vi "LabView SMART BABY CARE .vi"() -> ()   [LabVIEW 2020]
uses:
  <vilib>/Instr/_visa.llb/VISA Configure Serial Port (Instr).vi
  <vilib>/express/express analysis/Spectral/Block/exnSpectralBlock spectral measurements peak poly.vi
  <vilib>/express/express analysis/Spectral/Block/exnSpectralBlock spectral measurements peak DDT.vi
  <vilib>/httpClient/PUTBuffer.vi
  <vilib>/express/express analysis/Spectral/XNode/ExpressSpectralMeasurementsBlockNode.xnode
  <vilib>/httpClient/LabVIEWHTTPClient.lvlib
  <vilib>/ptbypt/NI_PtbyPt.lvlib
panel:
  out "reset signal":bool caption="Time has Elapsed"
  out "swing status":bool caption="Time has Elapsed"
  out "net status":bool caption="Time has Elapsed"
  out "fan status":bool caption="Time has Elapsed"
  out "fan speed":dbl
  out "temperture":dbl(knob) scale=15.0..50.0
  in  "VISA resource name":refnum<visa-resource-name>
  out "danger_movement":bool caption="Time has Elapsed"
  out "angle":dbl(knob) scale=-90.0..90.0
  out "vol-angle":dbl
  out "crying_sound":bool caption="Time has Elapsed"
  out "baby_present":bool
  out "lux":dbl
  out "volt lux":dbl
  out "volt wet":dbl
  out "wet":bool caption="Time has Elapsed"
  out "Waveform Graph":dynamicdata(graph)
  out "baby_crying":bool caption="Time has Elapsed"
  out "Amplitude of sound":dbl
  out "net comand":bool
  out "fan command":bool
  in  "stop":bool
  # "SMART BABY CARE SYSTEM"
  # "BY GROUP 05"
  # "BABY MONITORING AND CRY DETECT"
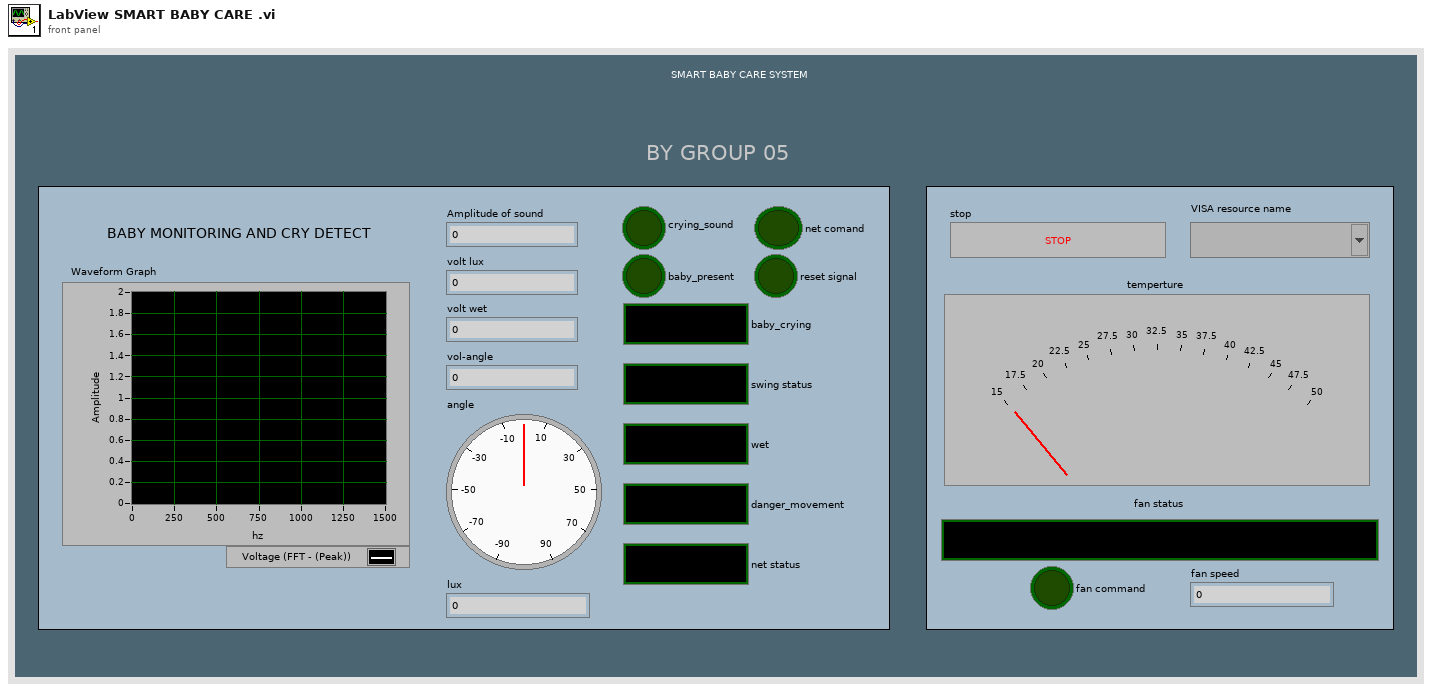
[diagram p1: front panel]
types:
  T1 = typedef "LabVIEWHTTPClient.lvlib/ClientHandle.ctl" = refnum<k1>
  T2 = cluster{"fan_command":bool, "net_command":bool, "net_adjust_time":string, "net_reset":bool}
  T3 = cluster{"averaging mode":u16, "weighting mode":u16, "number of averages":u32}
  T4 = cluster{"dB On (F)":bool, "unwrap phase (F)":bool, "convert to degree (F)":bool}
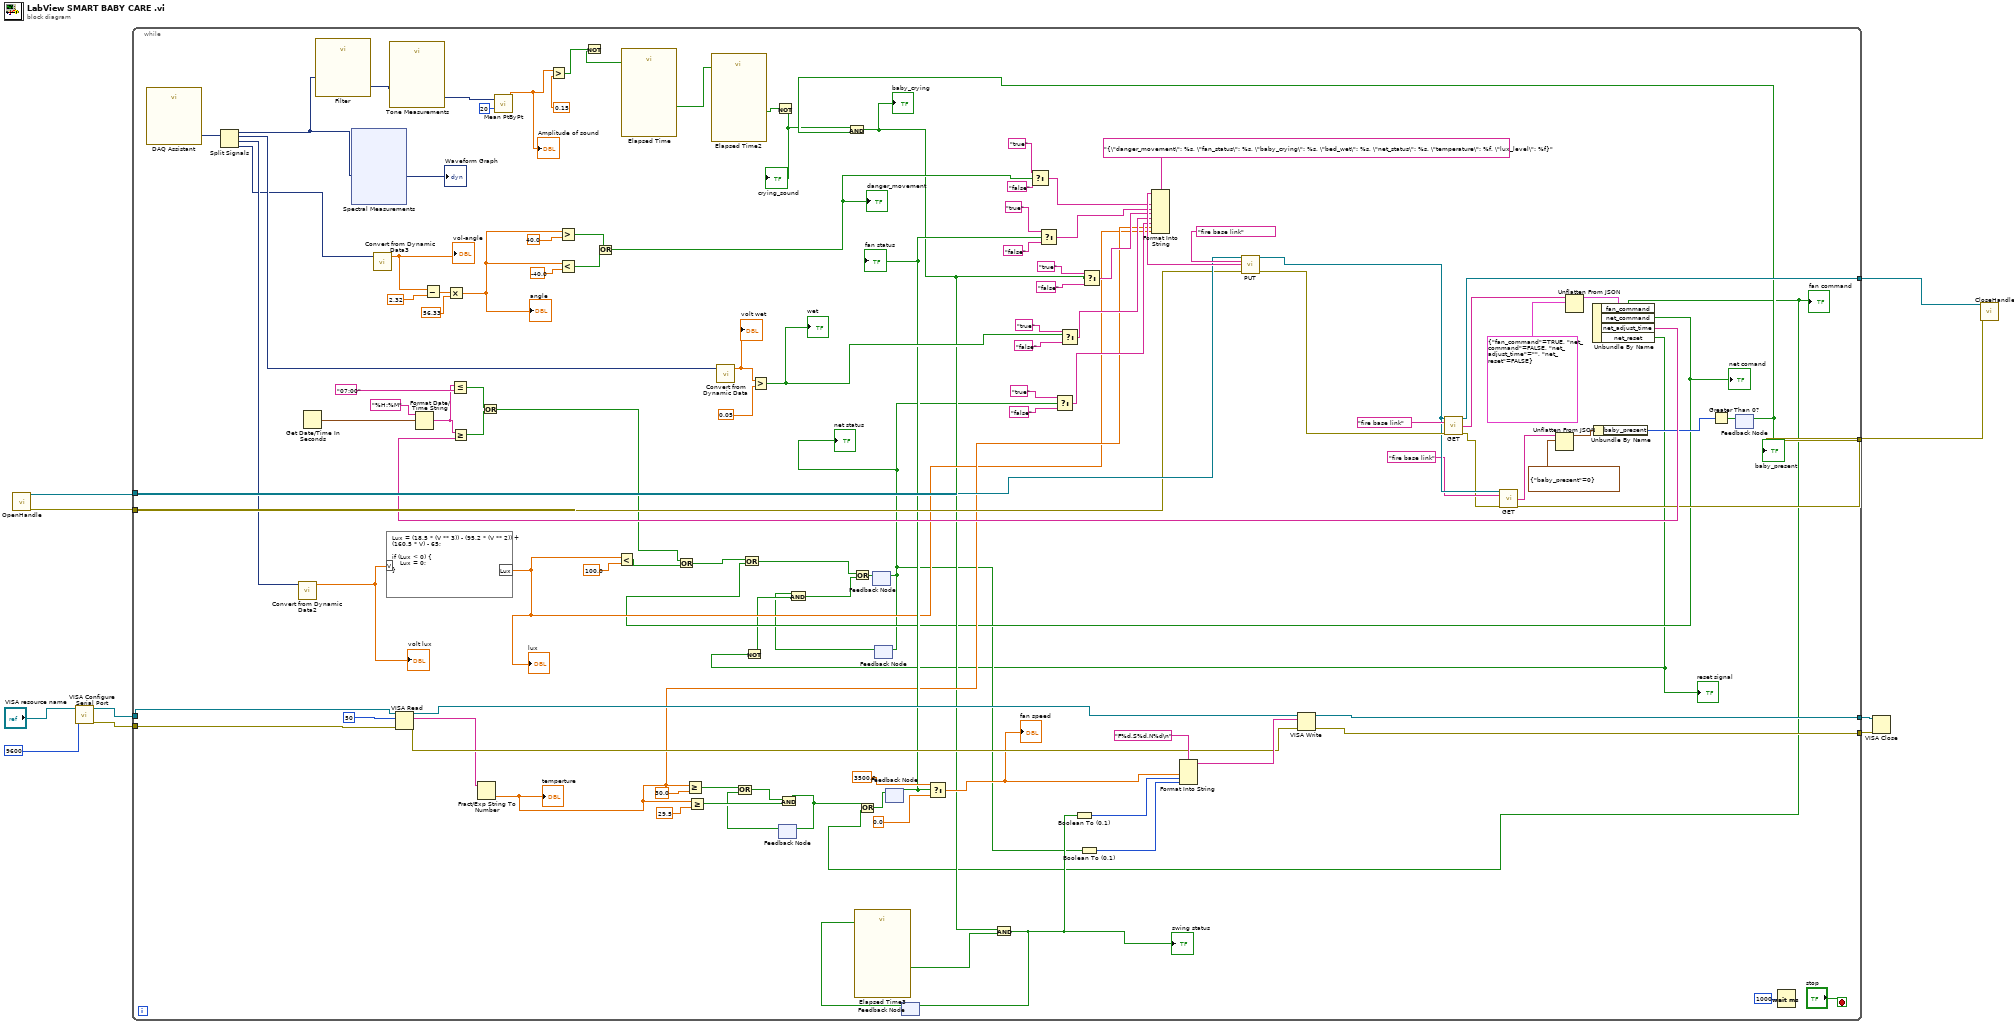
[diagram p0: block diagram]
diagram:
  n1 = call <vilib>:"OpenHandle.vi"() -> ("client handle out"=w10:T1, "error out"=w7:errorcluster)  [unwired: 14 in]
  n2 = call-poly "VISA Configure Serial Port"("VISA resource name"="VISA resource name", "baud rate (9600)"=u32 9600) -> ("VISA resource name out"=w4:refnum<visa-resource-name>, "error out"=w3:errorcluster)  [unwired: 12 in]
  n3 = while {
    tunnel: w10 -> [w107]
    tunnel: [w74] -> w9
    tunnel: [w72] -> w8
    tunnel: w7 -> [w105]
    tunnel: w4 -> [w47]
    tunnel: w3 -> [w48]
    tunnel: [w50] -> w2
    tunnel: [w49] -> w1
    stop <- "stop" stop-if-true
    n4 = call "DAQ Assistant"() -> ("data"=w82:dynamicdata)  [unwired: 17 in, 2 out]
    n5 = Split Signals(w82) -> (w81:dynamicdata, w80:dynamicdata, w78:dynamicdata, w15:dynamicdata)  [unwired: 4 in]
    n6 = call "Convert from Dynamic Data2"("Dynamic Data Type"=w78) -> ("Scalar"=w77:dbl)  [unwired: 3 in]
    "volt lux" <- w77
    n7 = Get Date/Time In Seconds() -> (seconds since 1Jan1904=w96:timestamp)
    n8 = call "Filter"("Signal"=w81) -> ("Filtered Signal"=w94:dynamicdata)  [unwired: 9 in, 1 out]
    n9 = xnode "Spectral Measurements"("Signals"=w81) -> ("FFT - (Peak)"=→"Waveform Graph":dynamicdata)  [unwired: 1 in, 2 out]
    n10 = call "Convert from Dynamic Data3"("Dynamic Data Type"=w15) -> ("Scalar"=w64:dbl)  [unwired: 3 in]
    "vol-angle" <- w64
    n11 = formula code="Lux = (18.5 * (V ** 3)) - (95.2 * (V ** 2)) + (160.5 * V) - 65;\n\nif (Lux < 0) {\n    Lux = 0;\n}"("V"=w77) -> ("Lux"=w31:dbl)
    "lux" <- w31
    n12 = call "Tone Measurements"("Signals"=w94) -> ("Amplitude"=w90:dynamicdata)  [unwired: 9 in, 1 out]
    n13 = VISA Read(VISA resource name=w47, byte count=u32 50, error in (no error)=w48) -> (VISA resource name out=w45:refnum<visa-resource-name>, read buffer=w40:string, error out=w46:errorcluster)  [unwired: 1 out]
    n14 = Format Date/Time String(time format string (%c)="%H:%M", seconds (now)=w96) -> (date/time string=w95:string)  [unwired: 1 in]
    n15 = Subtract(x=w64, y=2.32) -> (x-y=w62:dbl)
    n16 = Multiply(x=w62, y=56.33) -> (x*y=w58:dbl)
    "angle" <- w58
    n17 = Less Or Equal?(x=w95, y="07:00") -> (x <= y?=w99:bool)
    n18 = Fract/Exp String To Number(string=w40) -> (number=w33:dbl)  [unwired: 3 in, 1 out]
    "temperture" <- w33
    n19 = call <vilib>:"Mean PtByPt.vi"("x"=w90, "sample length"=20) -> ("mean"=w88:dbl)  [unwired: 2 in, 1 out]
    "Amplitude of sound" <- w88
    n20 = Greater?(x=w88, y=0.15) -> (0:w92:bool)
    n21 = Greater?(x=w58, y=40.0) -> (0:w57:bool)
    n22 = Less?(x=w58, y=-40.0) -> (x < y?=w56:bool)
    n23 = Not(x=w92) -> (.not. x?=w91:bool)
    n24 = Or(x=w57, y=w56) -> (x .or. y?=w55:bool)
    "danger_movement" <- w55
    n25 = Less?(x=w31, y=100.0) -> (x < y?=w24:bool)
    n26 = call "Elapsed Time"("Reset"=w91) -> ("Time has Elapsed"=w87:bool)  [unwired: 11 in, 7 out]
    n27 = Greater Or Equal?(x=w33, y=30.0) -> (x >= y?=w41:bool)
    n28 = Greater Or Equal?(x=w33, y=29.5) -> (x >= y?=w38:bool)
    n29 = call "Elapsed Time2"("Reset"=w87) -> ("Time has Elapsed"=w86:bool)  [unwired: 11 in, 7 out]
    n30 = call "Convert from Dynamic Data"("Dynamic Data Type"=w80) -> ("Scalar"=w79:dbl)  [unwired: 3 in]
    "volt wet" <- w79
    n31 = Greater?(x=w79, y=0.05) -> (0:w83:bool)
    "wet" <- w83
    n32 = Not(x=w86) -> (.not. x?=w65:bool)
    "crying_sound" <- w65
    n33 = feedback #1() -> (w37:bool)  [unwired: 1 in]
    n34 = Or(x=w41, y=w37) -> (x .or. y?=w39:bool)
    n35 = And(x=w39, y=w38) -> (x .and. y?=w12:bool)
    n36 = feedback-in #1(w12) -> ()
    n37 = feedback #2() -> (w16:bool)  [unwired: 1 in]
    "net status" <- w16
    n38 = feedback-in #3(w16) -> ()
    n39 = feedback #3() -> (w18:bool)  [unwired: 1 in]
    n40 = feedback #4() -> (w34:bool)  [unwired: 1 in]
    "fan status" <- w34
    n41 = feedback #5() -> (w27:bool)  [unwired: 1 in]
    n42 = call "Elapsed Time3"("Reset"=w27) -> ("Time has Elapsed"=w28:bool)  [unwired: 11 in, 7 out]
    n43 = Select(t=3500.0, s=w34, f=0.0) -> (s? t:f=w32:dbl)
    "fan speed" <- w32
    n44 = Select(t="true", s=w55, f="false") -> (s? t:f=w121:string)
    n45 = Select(t="true", s=w34, f="false") -> (s? t:f=w118:string)
    n46 = Select(t="true", s=w16, f="false") -> (s? t:f=w109:string)
    n47 = Select(t="true", s=w83, f="false") -> (s? t:f=w110:string)
    n48 = Boolean To (0,1)(Boolean=w16) -> (0, 1=w52:i16)
    n49 = feedback #6() -> (w66:bool)  [unwired: 1 in]
    "baby_present" <- w66
    n50 = And(x=w65, y=w66) -> (x .and. y?=w29:bool)
    "baby_crying" <- w29
    n51 = And(x=w29, y=w28) -> (x .and. y?=w26:bool)
    "swing status" <- w26
    n52 = feedback-in #5(w26) -> ()
    n53 = Boolean To (0,1)(Boolean=w26) -> (0, 1=w53:i16)
    n54 = Select(t="true", s=w29, f="false") -> (s? t:f=w115:string)
    n55 = Format Into String(format string="{\"danger_movement\": %s, \"fan_status\": %s, \"baby_crying\": %s, \"bed_wet\": %s, \"net_status\": %s, \"temperature\": %f, \"lux_level\": %f}", w121, w118, w115, w110, w109, w33, w31) -> (resulting string=w126:string)  [unwired: 2 in, 1 out]
    n56 = Format Into String(format string="F%d,S%d,N%d\n", w32, w53, w52) -> (resulting string=w51:string)  [unwired: 2 in, 1 out]
    n57 = call-poly <vilib>:"PUT.vi"("client handle"=w107, "url"="fire base link", "buffer"=w126, "error in (no error)"=w105) -> ("client handle out"=w76:T1, "error out"=w106:errorcluster)  [unwired: 8 in, 2 out]
    n58 = VISA Write(VISA resource name=w45, write buffer=w51, error in (no error)=w46) -> (VISA resource name out=w50:refnum<visa-resource-name>, error out=w49:errorcluster)  [unwired: 1 out]
    n59 = call <vilib>:"GET.vi"("client handle"=w76, "url"="fire base link", "error in (no error)"=w106) -> ("client handle out"=w74:T1, "body"=w104:string, "error out"=w73:errorcluster)  [unwired: 9 in, 1 out]
    n60 = call <vilib>:"GET.vi"("client handle"=w76, "url"="fire base link", "error in (no error)"=w73) -> ("body"=w71:string, "error out"=w72:errorcluster)  [unwired: 9 in, 2 out]
    n61 = Unflatten From JSON(JSON string=w71, type and defaults=cluster{"baby_present":i32} {"baby_present"=0}) -> (value=w69:cluster{"baby_present":i32})  [unwired: 5 in, 1 out]
    n62 = Unflatten From JSON(JSON string=w104, type and defaults=T2 {"fan_command"=TRUE, "net_command"=FALSE, "net_adjust_time"="", "net_reset"=FALSE}) -> (value=w102:T2)  [unwired: 5 in, 1 out]
    n63 = Unbundle By Name(w102) -> ("fan_command"=w13:bool, "net_command"=w22:bool, "net_adjust_time"=w101:string, "net_reset"=w11:bool)
    "fan command" <- w13
    "net comand" <- w22
    "reset signal" <- w11
    n64 = Greater Or Equal?(x=w95, y=w101) -> (x >= y?=w98:bool)
    n65 = Or(x=w99, y=w98) -> (x .or. y?=w25:bool)
    n66 = Or(x=w25, y=w24) -> (x .or. y?=w23:bool)
    n67 = Or(x=w23, y=w22) -> (x .or. y?=w20:bool)
    n68 = Not(x=w11) -> (.not. x?=w21:bool)
    n69 = And(x=w18, y=w21) -> (x .and. y?=w19:bool)
    n70 = Or(x=w20, y=w19) -> (x .or. y?=w17:bool)
    n71 = Or(x=w12, y=w13) -> (x .or. y?=w14:bool)
    n72 = feedback-in #2(w17) -> ()
    n73 = feedback-in #4(w14) -> ()
    n74 = Unbundle By Name(w69) -> ("baby_present"=w68:i32)
    n75 = Greater Than 0?(x=w68) -> (x > 0?=w67:bool)
    n76 = feedback-in #6(w67) -> ()
    n77 = Wait (ms)(milliseconds to wait=u32 1000) -> ()  [unwired: 1 out]
  }
  n78 = VISA Close(VISA resource name=w2, error in (no error)=w1) -> ()  [unwired: 1 out]
  n79 = call <vilib>:"CloseHandle.vi"("client handle"=w9, "error in (no error)"=w8) -> ()  [unwired: 13 in, 1 out]
